vi "保存数据.vi"(4 "版本信息":string[](array[string])) -> (0 "其他可选保存数据":T3, 1 "从板个数":dbl=1.0, 2 "保存时间输入(ms)":dbl=100.0, 3 "输入状态":bool, 5 "其他可选保存数据 3":T1)   [LabVIEW 2013]
panel:
  in  "其他可选保存数据 2":T1
  in  "存储表头语言选择":cluster{"English":bool, "中文":bool}={"English"=TRUE, "中文"=FALSE}
  in  "停止保存数据":bool
  out "接收":bool
  in  "VIC_Receive":refnum<vi>
  in  "停止":bool
  in  "VCI_Receive":T2 {"Rsv3" max=0 format="%x"; "Rsv2" min=101 format="%x"; "Rsv1" format="%x"; "Data8" format="%x"; "Data7" format="%x"; "Data6" format="%x"; "Data5" format="%x"; "Data4" format="%x"; "Data3" format="%x"; "Data2" format="%x"; "Data1" format="%x"; "DataLen" format="%x"; "ExternFlag" format="%x"; "RemoteFlag" format="%x"; "SendType" format="%x"; "TimeFlag" format="%x"; "TimeStamp" format="%x"; "ID" format="%x"}
  in  "获取版本信息":bool
  in  "退出":bool
  in  "确定":bool
  in  "从板个数":dbl=1.0
  in  "保存时间输入(ms)":dbl=500.0 format="%#.2f"
  in  "其他可选保存数据":T4
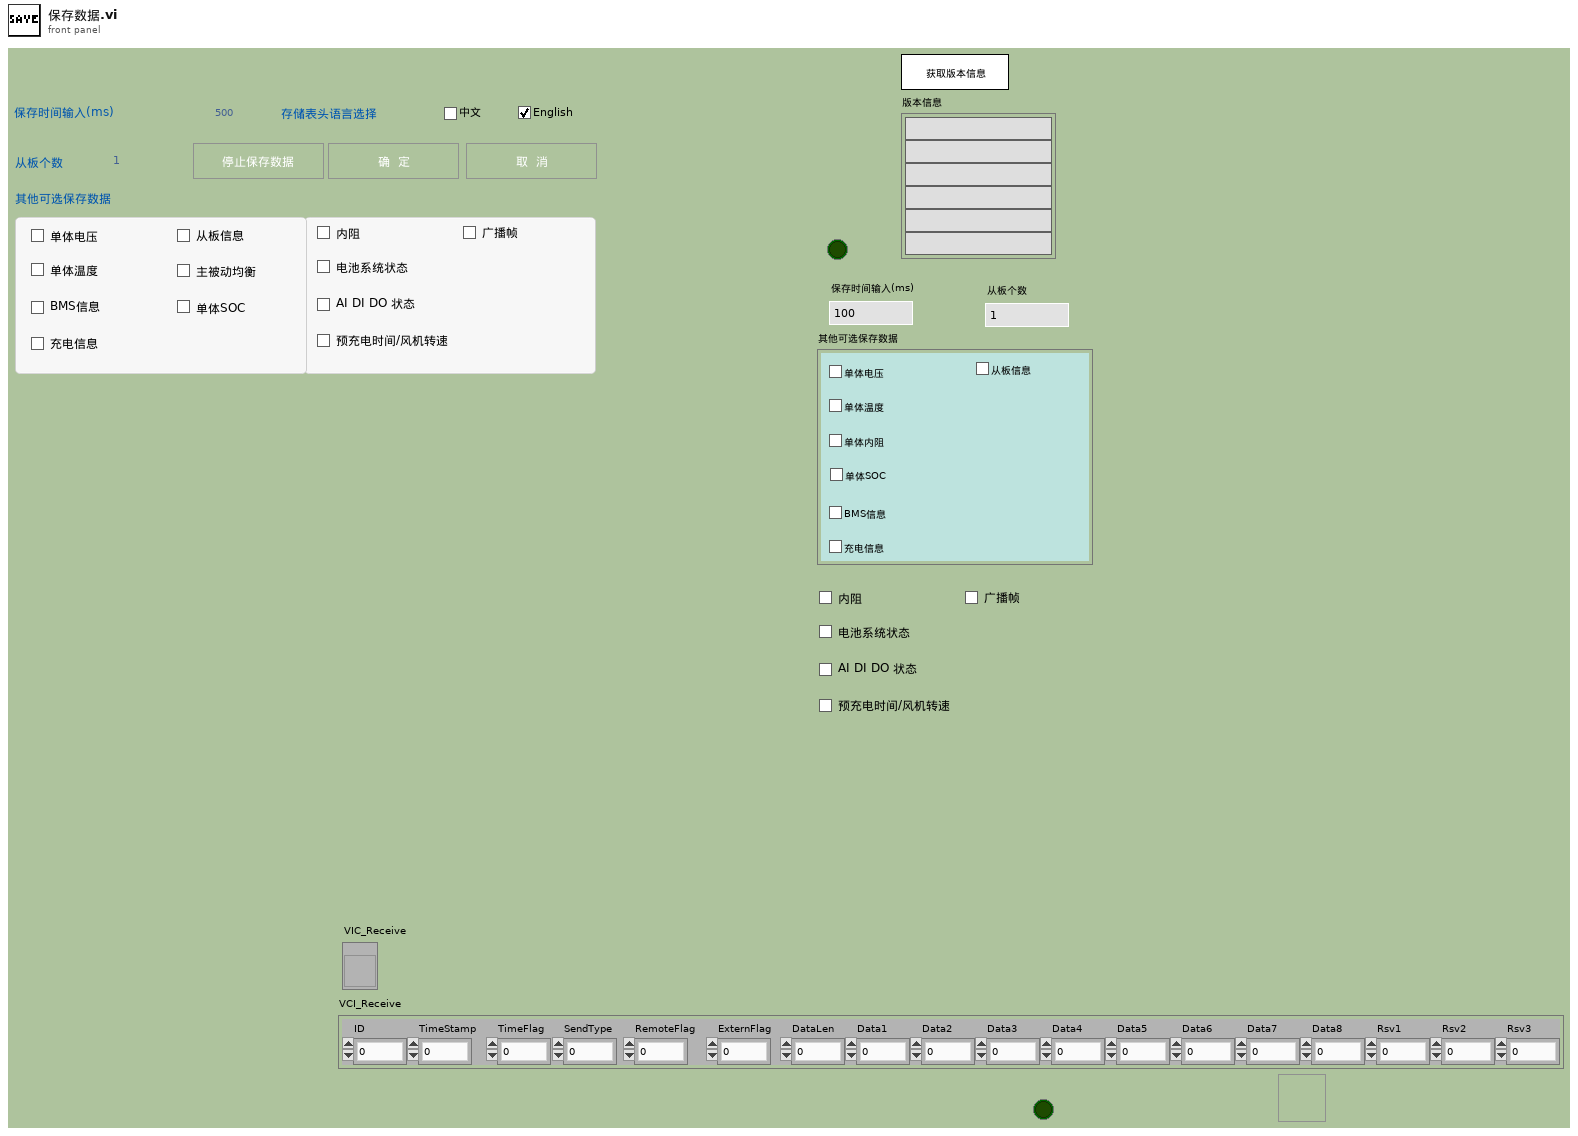
[diagram p1: front panel]
types:
  T1 = cluster{"单体电压":bool, "电池系统状态":bool, "AI DI DO 状态":bool, "预充电时间/风机转速":bool, "广播帧":bool}
  T2 = cluster{"ID":u32, "TimeStamp":u32, "TimeFlag":u8, "SendType":u8, "RemoteFlag":u8, "ExternFlag":u8, "DataLen":u8, "Data1":u8, "Data2":u8, "Data3":u8, "Data4":u8, "Data5":u8, "Data6":u8, "Data7":u8, "Data8":u8, "Rsv1":u8, "Rsv2":u8, "Rsv3":u8}
  T3 = cluster{"单体电压":bool, "单体温度":bool, "单体内阻":bool, "BMS信息":bool, "充电信息":bool, "从板信息":bool, "单体SOC":bool}
  T4 = cluster{"单体电压":bool, "单体温度":bool, "主被动均衡":bool, "BMS信息":bool, "充电信息":bool, "从板信息":bool, "单体SOC":bool}
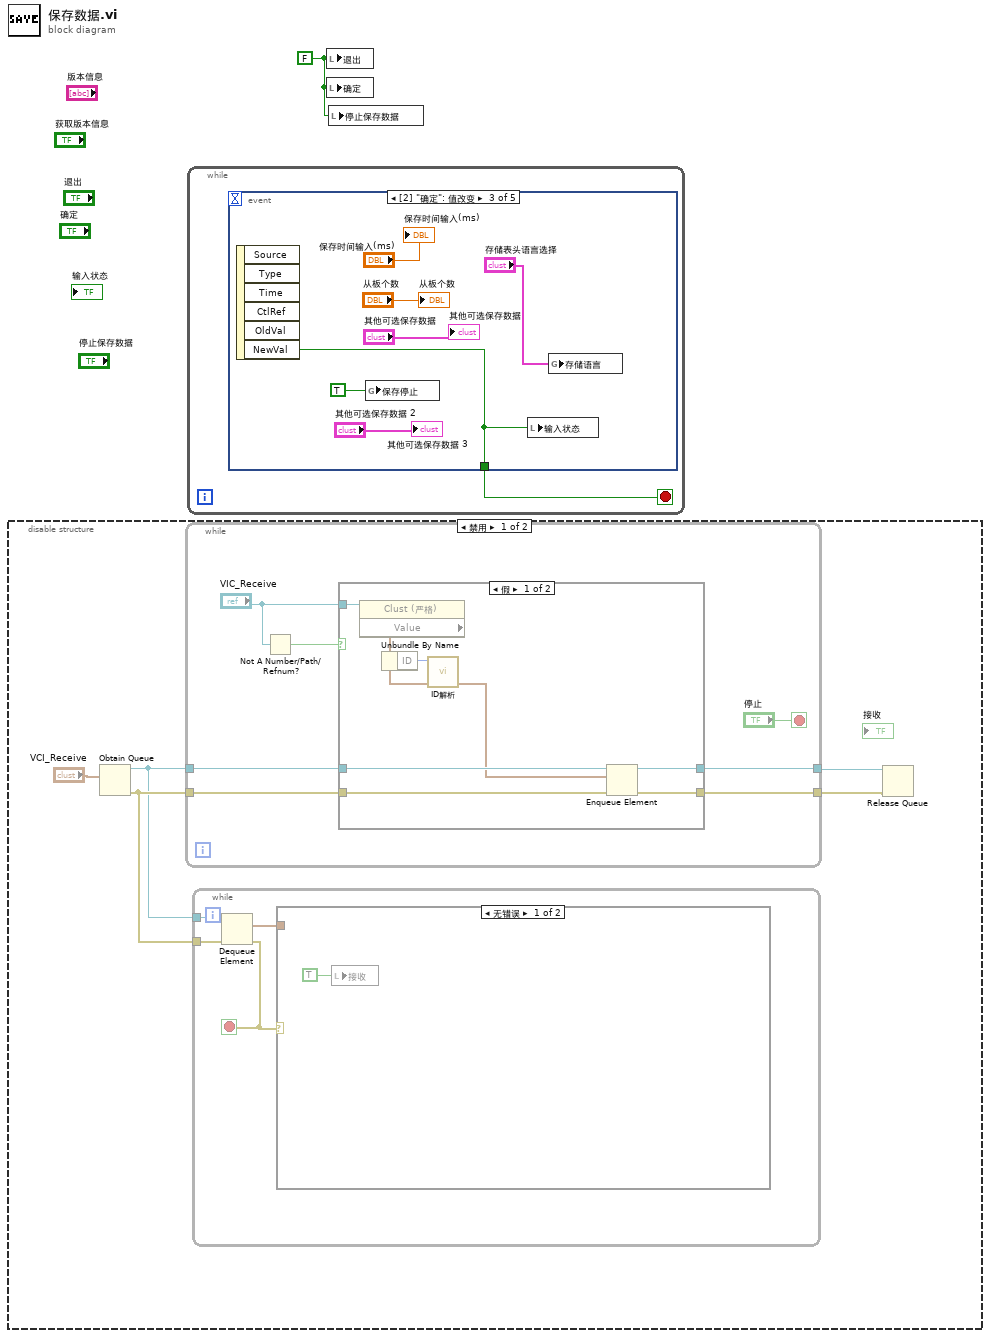
[diagram p0: block diagram]
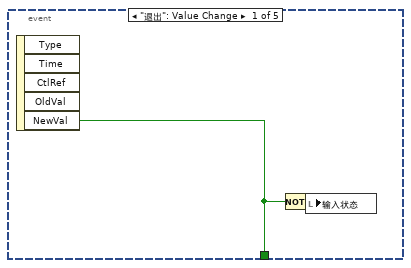
[diagram p5: hidden frame]
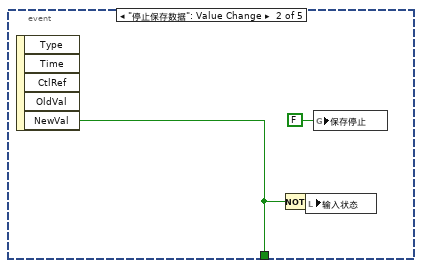
[diagram p6: hidden frame]
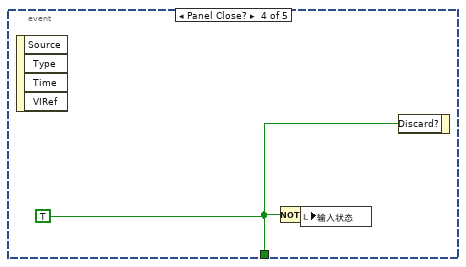
[diagram p7: hidden frame]
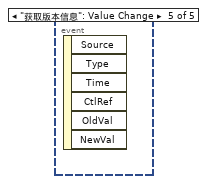
[diagram p8: hidden frame]
diagram:
  w1 = FALSE ("退出")
  n1 = disable-structure shown="禁用" {
    frame Disabled {
      n2 = Obtain Queue(element data type="VCI_Receive") -> (queue out=w5:refnum<queue>, error out=w6:errorcluster)  [unwired: 4 in, 1 out]
      n3 = while {
        tunnel: w5 -> [w16]
        tunnel: w6 -> [w15]
        tunnel: [w14] -> w3
        tunnel: [w13] -> w2
        stop <- "停止" stop-if-true
        n4 = Not A Number/Path/Refnum?(number/path/refnum="VIC_Receive") -> (NaN/Path/Refnum?=w12:bool)
        n5 = case shown="假" w12 {
          tunnel: w16 -> [w24 w27]
          tunnel: w15 -> [w23 w26]
          tunnel: [w21 w27] -> w14
          tunnel: [w20 w26] -> w13
          tunnel: "VIC_Receive" -> [w19 _]
          frame False {
            n6 = property class="Clust (严格)"(reference=w19) -> ("Value"=w22:T2)  [unwired: 1 in, 2 out]
            n7 = Unbundle By Name(w22) -> ("ID"=w25:u32)
            n8 = call "ID解析.vi"("ID"=w25) -> ()  [unwired: 11 out]
            n9 = Enqueue Element(queue=w24, element=w22, error in (no error)=w23) -> (queue out=w21:refnum<queue>, error out=w20:errorcluster)  [unwired: 2 out]
          }
          frame True {
          }
        }
      }
      n10 = while {
        tunnel: w5 -> [w9]
        tunnel: w6 -> [w8]
        stop <- w10 stop-if-true
        n11 = Dequeue Element(queue=w9, error in (no error)=w8) -> (element=w7:T2, error out=w10:errorcluster)  [unwired: 3 out]
        n12 = case shown="无错误" w10 {
          tunnel: w7 -> [_ _]
          frame No Error {
            n13 = local write "接收"(TRUE ("接收")) -> ()
          }
          frame Error {
          }
        }
      }
      n14 = Release Queue(queue=w3, error in (no error)=w2) -> ()  [unwired: 4 out]
    }
    frame Enabled {
    }
  }
  n15 = while {
    stop <- w28 stop-if-true
    n16 = event shown="[2] \"确定\": 值改变" {
      selector: _ -> [_ _ _ _ _]
      dyn-events: _ -> [_ _ _ _ _]
      timeout: _ -> [_ _ _ _ _]
      tunnel: [w29 w32 w40 w42 _] -> w28
      event "退出": Value Change {
        n17 = event-data() -> ("NewVal"=w29:bool)  [unwired: 5 out]
        n18 = Not(x=w29) -> (.not. x?=w30:bool)
        n19 = local write "输入状态"(w30) -> ()
      }
      event "停止保存数据": Value Change {
        n20 = event-data() -> ("NewVal"=w32:bool)  [unwired: 5 out]
        n21 = Not(x=w32) -> (.not. x?=w33:bool)
        n22 = local write "输入状态"(w33) -> ()
        n23 = global write "全局 1.vi" "保存停止"(FALSE ("保存停止")) -> ()
      }
      event "确定": Value Change {
        n24 = event-data() -> ("NewVal"=w40:bool)  [unwired: 6 out]
        n25 = global write "全局 1.vi" "保存停止"(TRUE ("保存停止")) -> ()
        n26 = local write "输入状态"(w40) -> ()
        n27 = global write "EV05全局变量1.vi" "存储语言"("存储表头语言选择") -> ()
        "保存时间输入(ms)" <- "保存时间输入(ms)"
        "从板个数" <- "从板个数"
        "其他可选保存数据" <- "其他可选保存数据"
        "其他可选保存数据 3" <- "其他可选保存数据 2"
      }
      event Panel Close? {
        w42 = TRUE
        n28 = event-data() -> ()  [unwired: 5 out]
        n29 = Not(x=w42) -> (.not. x?=w41:bool)
        n30 = local write "输入状态"(w41) -> ()
        n31 = event-data("Discard?"=w42) -> ()  [unwired: 1 in, 1 out]
      }
      event "获取版本信息": Value Change {
        n32 = event-data() -> ()  [unwired: 7 out]
      }
    }
  }
  n33 = local write "退出"(w1) -> ()
  n34 = local write "确定"(w1) -> ()
  n35 = local write "停止保存数据"(w1) -> ()
